vi "failUnlessXmlGeneratedCorrectly.vi"(4 "Convert EOL? (TRUE)":bool=TRUE, 5 "Encoding (none)":string, 6 "message (\"\")":string, 8 "error in":errorcluster, 9 "expected XML string":string, 10 "Input Data":variant, 11 "EasyXMLTest in":refnum<class "EasyXMLTest.lvclass">) -> (0 "error out":errorcluster, 2 "Generated XML String":string, 3 "EasyXMLTest out":refnum<class "EasyXMLTest.lvclass">)   [LabVIEW 2013, in "EasyXMLTest.lvclass"]
uses:
  EasyXMLTest.lvclass
panel:
  # "Copyright © 2007 James Kring, Inc. All rights reserved.\n\nAuthor: Jim Kring [jim.kring@jameskring.com]\n\nThis library is provided \"AS IS\" ,WITHOUT WARRANTIES OR \nCONDITIONS OF ANY KIND, either express or implied.\n\nJames Kring, Inc. -- http://www.jameskring.com"
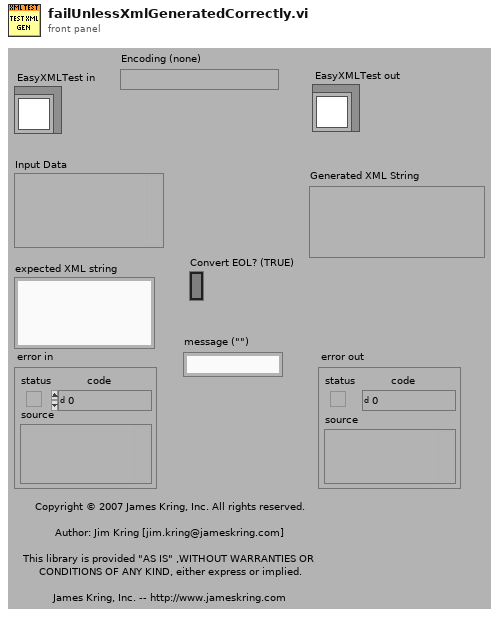
[diagram p1: front panel]
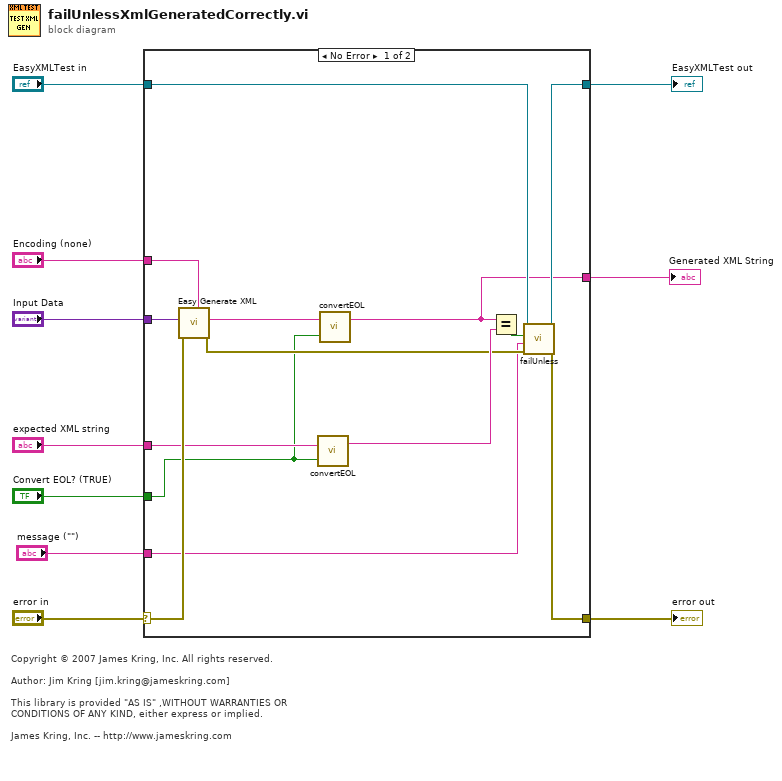
[diagram p0: block diagram]
diagram:
  # "Copyright © 2007 James Kring, Inc. All rights reserved.\n\nAuthor: Jim Kring [jim.kring@jameskring.com]\n\nThis library is provided \"AS IS\" ,WITHOUT WARRANTIES OR \nCONDITIONS OF ANY KIND, either express or implied.\n\nJames Kring, Inc. -- http://www.jameskring.com"
  n1 = case shown="No Error" "error in" {
    selector: "error in" -> [w23 w26]
    tunnel: [w18 w26] -> w5
    tunnel: "EasyXMLTest in" -> [w20 w25]
    tunnel: [w19 w25] -> w7
    tunnel: "Input Data" -> [w24 _]
    tunnel: "expected XML string" -> [w22 _]
    tunnel: "message (\"\")" -> [w15 _]
    tunnel: [w12 _] -> w3
    tunnel: "Convert EOL? (TRUE)" -> [w14 _]
    tunnel: "Encoding (none)" -> [w11 _]
    frame No Error {
      n2 = call "Easy Generate XML.vi"("Encoding (none)"=w11, "error in (no error)"=w23, "LabVIEW Data"=w24) -> ("error out"=w17:errorcluster, "XML String"=w13:string)  [unwired: 7 in]
      n3 = call "convertEOL.vi"("Convert EOL? (TRUE)"=w14, "string"=w22) -> ("string out"=w21:string)  [unwired: 1 in]
      n4 = call "convertEOL.vi"("Convert EOL? (TRUE)"=w14, "string"=w13) -> ("string out"=w12:string)  [unwired: 1 in]
      n5 = Equal?(x=w12, y=w21) -> (x = y?=w16:bool)
      n6 = call-dynamic "failUnless.vi"("error in (no error)"=w17, "message (\"\")"=w15, "pass"=w16, "TestCase in"=w20) -> ("error out"=w18:errorcluster, "TestCase out"=w19:refnum<class "EasyXMLTest.lvclass">)  [unwired: 6 in]
    }
    frame Error {
    }
  }
  "EasyXMLTest out" <- w7
  "error out" <- w5
  "Generated XML String" <- w3
